vi "subbus_read.vi"(8 "error in (no error)":errorcluster, 9 "PortIn":string, 11 "Address":u16 format="%x") -> (0 "error out":errorcluster, 1 "PortOut":string, 2 "Ack":bool, 3 "Data":u16 format="%x")   [LabVIEW 2016]
uses:
  <vilib>/Utility/error.llb/Error Cluster From Error Code.vi
  <vilib>/ErrorRing/Error Ring.xnode
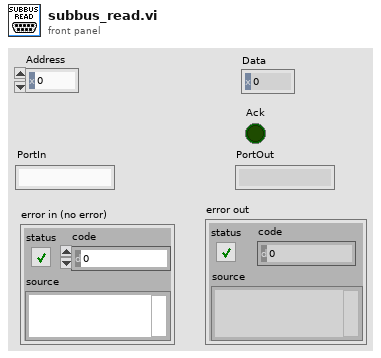
[diagram p1: front panel]
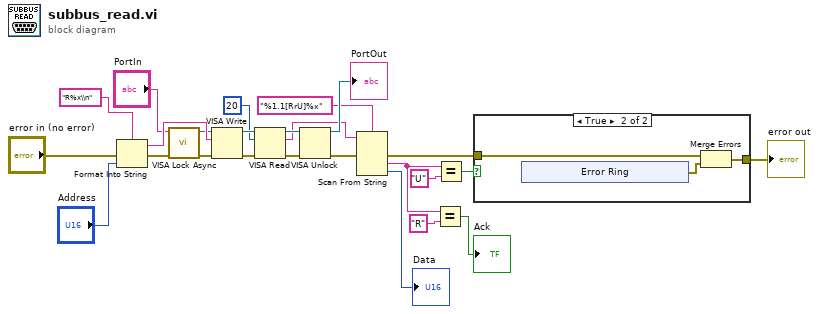
[diagram p0: block diagram]
diagram:
  n1 = Format Into String(format string="R%x\\n", error in="error in (no error)", "Address") -> (resulting string=w22:string, error out=w17:errorcluster)  [unwired: 1 in]
  n2 = call <vilib>:"VISA Lock Async.vi"("error in (no error)"=w17, "VISA resource name"="PortIn") -> ("error out"=w16:errorcluster, "VISA resource name out"=w15:refnum<visa-resource-name>)  [unwired: 7 in, 1 out]
  n3 = VISA Write(VISA resource name=w15, write buffer=w22, error in (no error)=w16) -> (VISA resource name out=w21:refnum<visa-resource-name>, error out=w20:errorcluster)  [unwired: 1 out]
  n4 = VISA Read(VISA resource name=w21, byte count=20, error in (no error)=w20) -> (VISA resource name out=w14:refnum<visa-resource-name>, read buffer=w10:string, error out=w13:errorcluster)  [unwired: 1 out]
  n5 = VISA Unlock(8:w13, 11:w14) -> (0:w9:errorcluster, 3:→"PortOut":refnum<visa-resource-name>)
  n6 = Scan From String(format string="%1.1[RrU]%x", input string=w10, error in=w9) -> (error out=w2:errorcluster, output 1=w5:string, output 2=→"Data":u16)  [unwired: 3 in, 2 out]
  n7 = Equal?(x=w5, y="R") -> (x = y?=→"Ack":bool)
  n8 = Equal?(x=w5, y="U") -> (x = y?=w3:bool)
  n9 = case shown="True" w3 {
    tunnel: w2 -> [w26 w29]
    tunnel: [w26 w27] -> w1
    frame False {
    }
    frame True {
      n10 = xnode "Error Ring"() -> ("error out"=w28:errorcluster)
      n11 = Merge Errors(w29, w28) -> (w27:errorcluster)
    }
  }
  "error out" <- w1
